vi "Bundle Script_In Place Remove Unwired.vi"(8 "error in":errorcluster, 11 "Affected Items":T1) -> (0 "error out":errorcluster)   [LabVIEW 2023]
doc: "Remove elements from In Place cluster bundler."
uses:
  top/BundleMagic.ctl
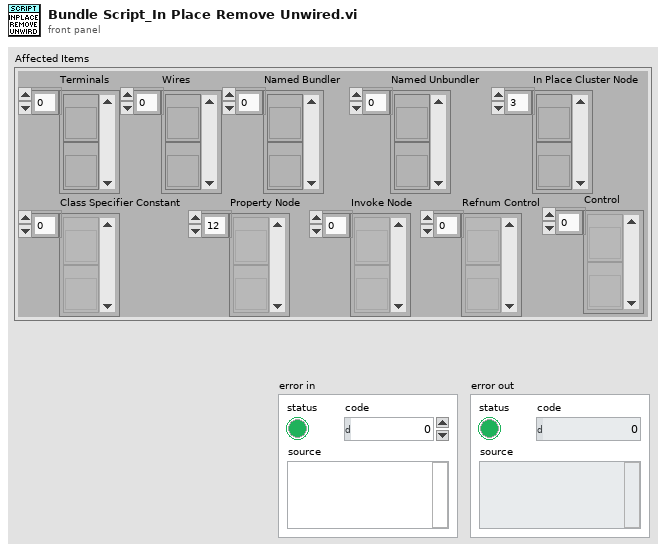
[diagram p1: front panel]
types:
  T1 = typedef "BundleMagic.ctl" = cluster{"Terminals":refnum<vi>[], "Wires":refnum<vi>[], "Named Bundler":refnum<vi>[], "Named Unbundler":refnum<vi>[], "In Place Cluster Node":refnum<vi>[], "Class Specifier Constant":refnum<vi>[], "Property Node":refnum<vi>[], "Invoke Node":refnum<vi>[], "Refnum Control":refnum<vi>[], "Control":refnum<vi>[]}
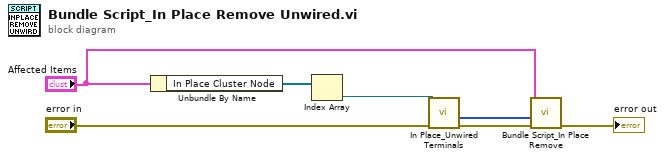
[diagram p0: block diagram]
diagram:
  n1 = Unbundle By Name("Affected Items") -> ("In Place Cluster Node"=w7:refnum<vi>[])
  n2 = Index Array(array=w7) -> (element=w5:refnum<vi>)  [unwired: 1 in]
  n3 = call "In Place_Unwired Terminals.vi"("error in"="error in", "In Place Node"=w5) -> ("error out"=w2:errorcluster, "Unwired Indices For Removal"=w3:u32[])  [unwired: 5 in, 3 out]
  n4 = call "Bundle Script_In Place Remove.vi"("error in"=w2, "Selected Item Indices"=w3, "Affected Items"="Affected Items") -> ("error out"=→"error out":errorcluster)  [unwired: 8 in]
